vi "Updating.vi"(8 "error in (no error)":errorcluster, 11 "Function in":refnum<class "Function.lvclass">) -> (0 "error out":errorcluster, 3 "Function out":refnum<class "Function.lvclass">)   [LabVIEW 2016, in "Function Actor.lvlib" / "Function.lvclass"]
uses:
  <userlib>/Common Components/Function Actor/Function.lvclass
  <userlib>/Common Components/Function Actor/Function.lvclass/Function.ctl
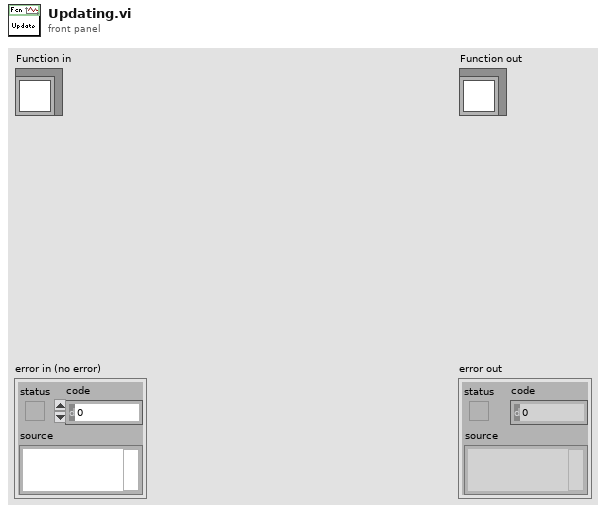
[diagram p1: front panel]
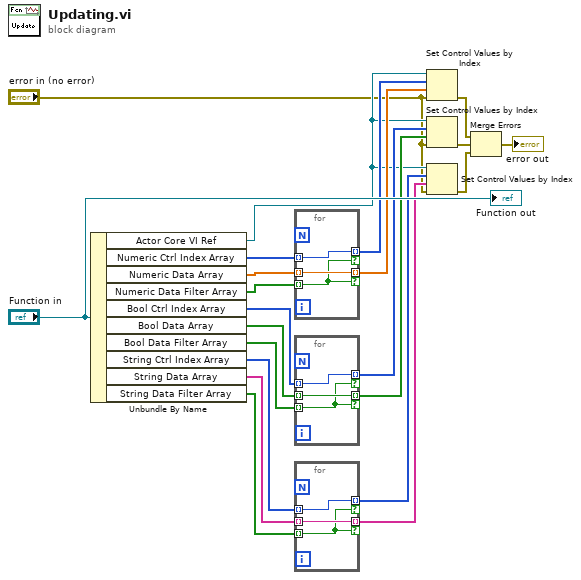
[diagram p0: block diagram]
diagram:
  n1 = Unbundle By Name("Function in") -> ("Actor Core VI Ref"=w5:refnum<vi>, "Numeric Ctrl Index Array"=w18:i32[], "Numeric Data Array"=w17:dbl[], "Numeric Data Filter Array"=w16:bool[], "Bool Ctrl Index Array"=w13:i32[], "Bool Data Array"=w12:bool[], "Bool Data Filter Array"=w9:bool[], "String Ctrl Index Array"=w8:i32[], "String Data Array"=w7:string[], "String Data Filter Array"=w6:bool[])
  n2 = for {
    tunnel: w18 -> [w25] mode=indexing
    tunnel: w17 -> [w24] mode=indexing
    tunnel: w16 -> [w23] mode=indexing
    tunnel: [w25] -> w15 mode=indexing if=w23
    tunnel: [w24] -> w14 mode=indexing if=w23
  }
  n3 = for {
    tunnel: w13 -> [w28] mode=indexing
    tunnel: w12 -> [w27] mode=indexing
    tunnel: w9 -> [w26] mode=indexing
    tunnel: [w28] -> w11 mode=indexing if=w26
    tunnel: [w27] -> w10 mode=indexing if=w26
  }
  n4 = for {
    tunnel: w8 -> [w31] mode=indexing
    tunnel: w7 -> [w30] mode=indexing
    tunnel: w6 -> [w29] mode=indexing
    tunnel: [w31] -> w4 mode=indexing if=w29
    tunnel: [w30] -> w3 mode=indexing if=w29
  }
  n5 = Set Control Values by Index(0:w5, 1:w15, 2:w14, 3:"error in (no error)") -> (11:w21:errorcluster)
  n6 = Set Control Values by Index(0:w5, 1:w11, 2:w10, 3:"error in (no error)") -> (11:w20:errorcluster)
  n7 = Set Control Values by Index(0:w5, 1:w4, 2:w3, 3:"error in (no error)") -> (11:w1:errorcluster)
  n8 = Merge Errors(w21, w20, w1) -> (→"error out":errorcluster)
  "Function out" <- "Function in"
